vi "Global Shutter.vi"() -> ()   [LabVIEW 2021]
panel:
  out "Error Out":errorcluster
  in  "VISA Refnum out":refnum<visa-resource-name>
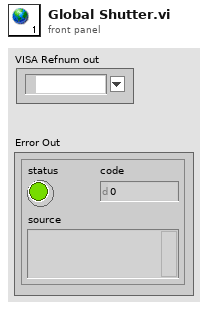
[diagram p1: front panel]
diagram:
